vi "MongoDB.SimpleExample3.vi"() -> ()   [LabVIEW 2014]
uses:
  Controls/Doc_TypeDef.ctl
  <vilib>/Analysis/baseanly.llb/Mean (DBL).vi
  MongoDB.Collection.lvclass
  MongoDB.Client.lvclass
  MongoDB.Database.lvclass
  <vilib>/Analysis/NI_AALBase.lvlib
panel:
  in  "error in (no error)":errorcluster
  out "error out":errorcluster
  in  "collectionName":string="testcollection1"
  in  "databaseName":string="labview_test"
  in  "connectionString":string="mongodb://labview_user:labview@ds045031.mongolab.com:45031/labview_test"
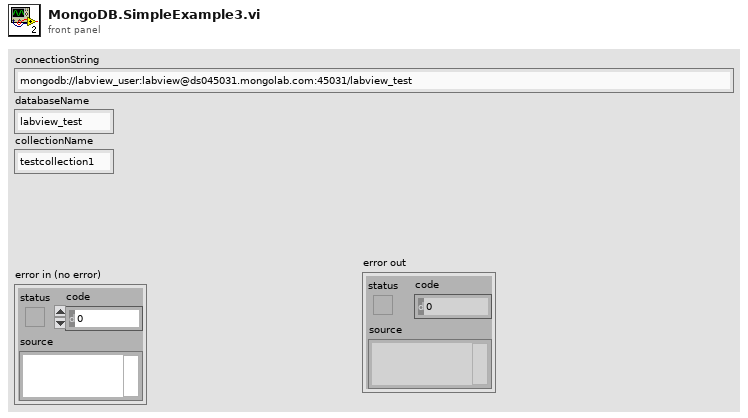
[diagram p1: front panel]
types:
  T1 = typedef "Doc_TypeDef.ctl" = cluster{"String":string, "I64":i64, "Bool":bool, "Dbl_Array":dbl[]}
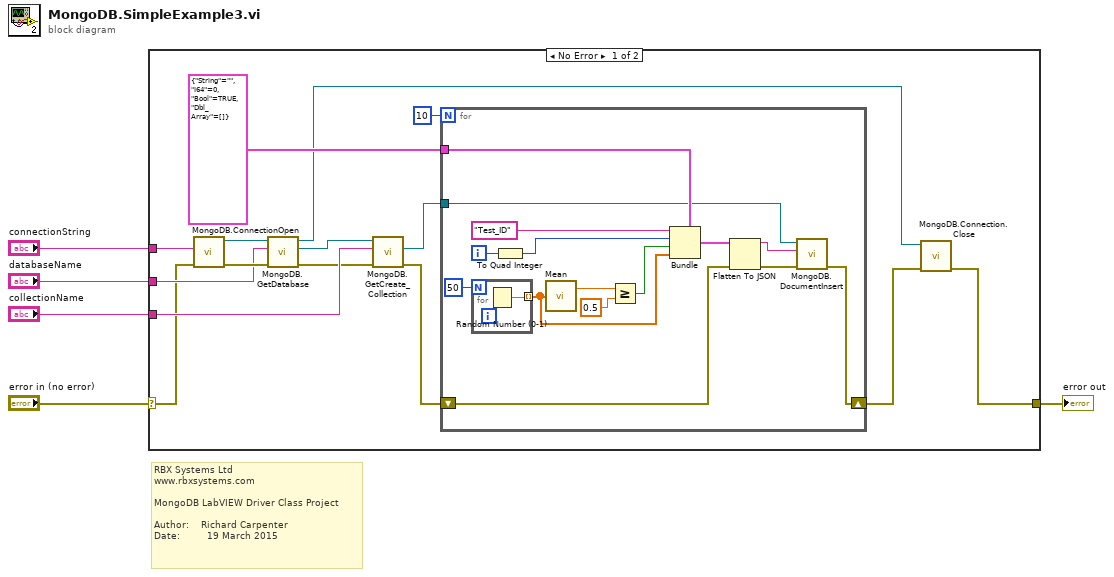
[diagram p0: block diagram]
diagram:
  # "RBX Systems Ltd\nwww.rbxsystems.com\n\nMongoDB LabVIEW Driver Class Project\n\nAuthor:    Richard Carpenter\nDate:         19 March 2015"
  n1 = case shown="No Error" "error in (no error)" {
    selector: "error in (no error)" -> [w13 w37]
    tunnel: "databaseName" -> [w18 _]
    tunnel: "connectionString" -> [w17 _]
    tunnel: "collectionName" -> [w15 _]
    tunnel: [w7 w37] -> w2
    frame No Error {
      n2 = call "MongoDB.ConnectionOpen.vi"("error in (no error)"=w13, "connectionString"=w17) -> ("error out"=w19:errorcluster, "MongoDB out"=w20:refnum<class "MongoDB.Client.lvclass">)  [unwired: 8 in]
      n3 = call "MongoDB.GetDatabase.vi"("error in (no error)"=w19, "databaseName"=w18, "MongoDB.Connection in"=w20) -> ("error out"=w14:errorcluster, "MongoDB.Database out"=w16:refnum<class "MongoDB.Database.lvclass">, "MongoDB.Connection out"=w9:refnum<class "MongoDB.Client.lvclass">)  [unwired: 6 in]
      n4 = call "MongoDB.GetCreate_Collection.vi"("error in (no error)"=w14, "collectionName"=w15, "MongoDB.Database in"=w16) -> ("error out"=w11:errorcluster, "MongoDB.Collection out"=w10:refnum<class "MongoDB.Collection.lvclass">)  [unwired: 6 in, 1 out]
      n5 = for {
        N: 10 -> [_]
        tunnel: T1 {"String"="", "I64"=0, "Bool"=TRUE, "Dbl_Array"=[]} -> [w35]
        tunnel: w10 -> [w23]
        shift-right: [w22] -> w8
        shift-left: w11 -> [w26]
        i -> [w33]
        n6 = for {
          N: 50 -> [_]
          tunnel: [w36] -> w28 mode=indexing
          n7 = Random Number (0-1)() -> (number: 0 to 1=w36:dbl)
        }
        n8 = To Quad Integer(1:w33) -> (0:w32:i64)
        n9 = call-poly <vilib>:"Mean.vi"("X"=w28) -> ("mean"=w30:dbl)  [unwired: 1 out]
        n10 = Greater Or Equal?(x=w30, y=0.5) -> (x >= y?=w29:bool)
        n11 = Bundle(cluster=w35, "String"="Test_ID", "I64"=w32, "Bool"=w29, "Dbl_Array"=w28) -> (w27:T1)
        n12 = Flatten To JSON(anything=w27, error in (no error)=w26) -> (JSON string=w24:string, 11:w25:errorcluster)  [unwired: 1 in]
        n13 = call-dynamic "MongoDB.DocumentInsert.vi"("error in (no error)"=w25, "JSON Document"=w24, "MongoDB.Collection in"=w23) -> ("error out"=w22:errorcluster)  [unwired: 6 in, 2 out]
      }
      n14 = call "MongoDB.Connection.Close.vi"("error in (no error)"=w8, "MongoDB in"=w9) -> ("error out"=w7:errorcluster)  [unwired: 9 in]
    }
    frame Error {
    }
  }
  "error out" <- w2
